vi "WaitForBrowser.vi"(4 "Send Command":bool=TRUE, 6 "BrowserCommand":string, 8 "Error In":errorcluster, 9 "Interval":dbl=0.1, 10 "Seconds":dbl=1.0, 11 "BrowserRef":refnum<k7>) -> (0 "Error Out":errorcluster, 3 "BrowserRefOut":refnum<k7>)   [LabVIEW 2010]
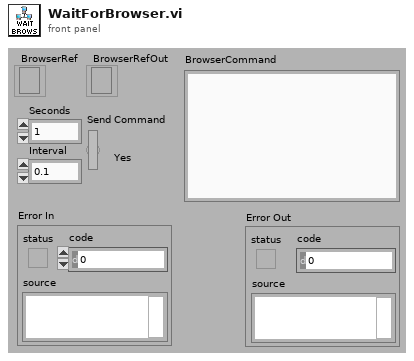
[diagram p1: front panel]
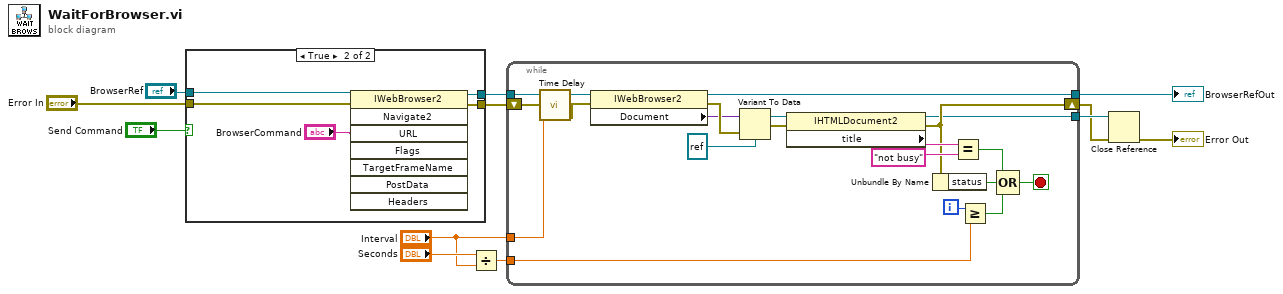
[diagram p0: block diagram]
diagram:
  n1 = case shown="True" "Send Command" {
    tunnel: [w14 w18] -> w10
    tunnel: [w13 w17] -> w9
    tunnel: "Error In" -> [w13 w16]
    tunnel: "BrowserRef" -> [w14 w15]
    frame False {
    }
    frame True {
      n2 = invoke class="IWebBrowser2" method="Navigate2"(reference=w15, error in=w16, "URL"="BrowserCommand") -> (reference out=w18:refnum<k7>, error out=w17:errorcluster)  [unwired: 5 in, 6 out]
    }
  }
  n3 = Divide(x="Seconds", y="Interval") -> (x/y=w12:dbl)
  n4 = while {
    tunnel: w10 -> [w29]
    tunnel: "Interval" -> [w20]
    tunnel: w12 -> [w35]
    shift-right: [w24] -> w6
    shift-left: w9 -> [w22]
    tunnel: [w28] -> w8
    tunnel: [w23] -> w7
    i -> [w39]
    stop <- w36 stop-if-true
    n5 = call "Time Delay"("error in (no error)"=w22, "Delay Time (s)"=w20) -> ("error out"=w21:errorcluster)  [unwired: 9 in]
    n6 = property class="IWebBrowser2"(reference=w29, error in=w21) -> (reference out=w28:refnum<k7>, error out=w31:errorcluster, "Document"=w30:variant)
    n7 = Variant To Data(error in=w31, Variant=w30, type=refnum<k7> refnum ("WebBrowser")) -> (error out=w34:errorcluster, data=w33:refnum<k7>)
    n8 = property class="IHTMLDocument2"(reference=w33, error in=w34) -> (reference out=w23:refnum<k7>, error out=w24:errorcluster, "title"=w27:string)
    n9 = Unbundle By Name(w24) -> ("status"=w38:bool)
    n10 = Equal?(x=w27, y="not busy") -> (x = y?=w25:bool)
    n11 = Greater Or Equal?(x=w39, y=w35) -> (x >= y?=w37:bool)
    n12 = Compound Arithmetic op=OR(w25, w38, w37) -> (w36:bool)
  }
  "BrowserRefOut" <- w8
  n13 = Close Reference(reference=w7, error in (no error)=w6) -> (error out=→"Error Out":errorcluster)
